vi "create_log.vi"(0 "Action":u16, 1 "Read Value":dbl, 2 "VISA resource name":refnum<visa-resource-name>, 3 "Volume Dispensed":string, 4 "Lower Threshold":dbl, 6 "Upper Threshold":dbl) -> (5 "Output Array":string[](array[string]))   [LabVIEW 2019]
uses:
  <vilib>/Utility/file.llb/Write Delimited Spreadsheet (string).vi
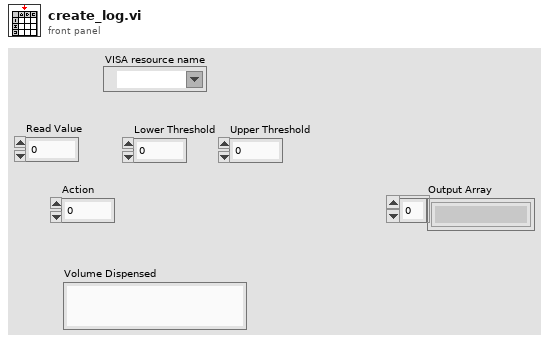
[diagram p1: front panel]
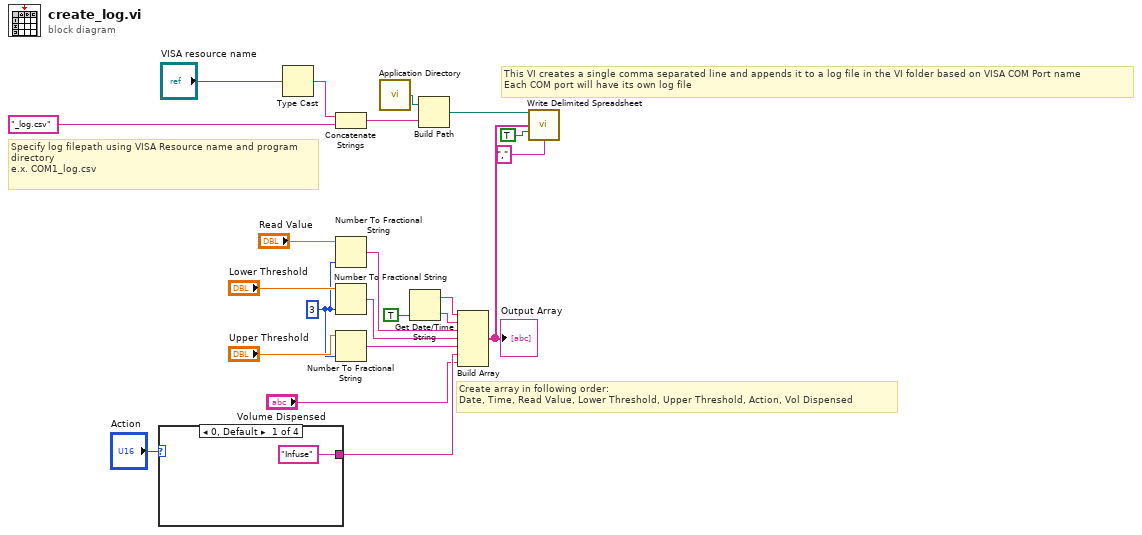
[diagram p0: block diagram]
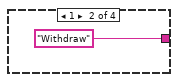
[diagram p2: hidden frame]
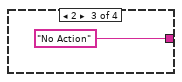
[diagram p3: hidden frame]
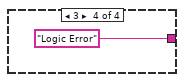
[diagram p4: hidden frame]
diagram:
  w2 = 3
  # "This VI creates a single comma separated line and appends it to a log file in the VI folder based on VISA COM Port name\nEach COM port will have its own log file"
  # "Create array in following order:\nDate, Time, Read Value, Lower Threshold, Upper Threshold, Action, Vol Dispensed"
  # "Specify log filepath using VISA Resource name and program directory\ne.x. COM1_log.csv"
  n1 = case shown="0, Default" "Action" {
    tunnel: ["Infuse" "Withdraw" "No Action" "Logic Error"] -> w3
    frame 0, Default {
    }
    frame 1 {
    }
    frame 2 {
    }
    frame 3 {
    }
  }
  n2 = Type Cast(x="VISA resource name") -> (*(type *) &x=w16:string)  [unwired: 1 in]
  n3 = Concatenate Strings(w16, "_log.csv" ("string")) -> (w14:string)
  n4 = Number To Fractional String(number="Read Value", precision (6)=w2) -> (F-format string=w9:string)  [unwired: 2 in]
  n5 = Number To Fractional String(number="Lower Threshold", precision (6)=w2) -> (F-format string=w5:string)  [unwired: 2 in]
  n6 = Number To Fractional String(number="Upper Threshold", precision (6)=w2) -> (F-format string=w6:string)  [unwired: 2 in]
  n7 = call <vilib>:"Application Directory.vi"() -> ("Application Directory"=w13:path)
  n8 = Get Date/Time String(want seconds? (F)=TRUE) -> (date string=w11:string, time string=w10:string)  [unwired: 2 in]
  n9 = Build Path(base path=w13, name or relative path=w14) -> (appended path=w17:path)
  n10 = Build Array(w11, w10, w9, w5, w6, w3, "Volume Dispensed") -> (w18:string[])
  "Output Array" <- w18
  n11 = call-poly <vilib>:"Write Delimited Spreadsheet.vi"("file path (dialog if empty)"=w17, "1D data"=w18, "append to file? (new file:F)"=TRUE, "delimiter (\\t)"="," ("delimiter (\\t)")) -> ()  [unwired: 10 in, 2 out]
